vi "LINC Standard Callback.vi"(2 "command in":string, 3 "target name":string) -> (0 "command out":string, 1 "GUID":string)   [LabVIEW 2018, in "STEPkgDriver_LINC.lvlib"]
uses:
  STEPkgDriver_LINC.lvlib
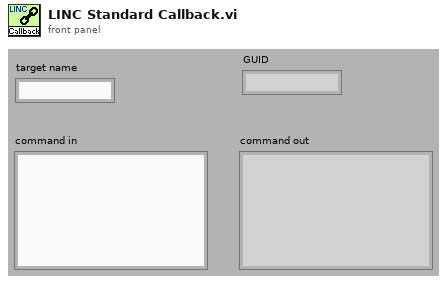
[diagram p1: front panel]
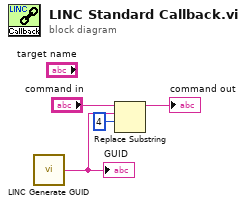
[diagram p0: block diagram]
diagram:
  n1 = call "LINC Generate GUID.vi"() -> ("GUID"=w1:string)
  "GUID" <- w1
  n2 = Replace Substring(3:4 ("offset (0)"), 4:w1, 5:"command in") -> (1:→"command out":string)  [unwired: 2 out]
